vi "Temperature Device (Set).vi"(6 "ISOBUS address":T10=-1 caption="ISOBUS address (-1)", 8 "error in":errorcluster, 10 "Temperature Device Settings":T3, 11 "Mercury Reference In":T11) -> (0 "error out":errorcluster, 2 "Response":T1, 3 "Mercury Reference Out":T11, 4 "Valid?":T2)   [LabVIEW 2013, in "Mercury iXX.lvlib" / "Temperature.lvlib"]
doc: "Set the temperature device configuration."
uses:
  Temperature.lvlib
  Mercury iXX.lvlib
  Private/Controls/Command Verbs.ctl
  Controls/Is Valid LED.ctl
  Controls/Comms Transport Layer.ctl
  Controls/Mercury Reference.ctl
  Controls/Excitation Type.ctl
  Controls/Response String.ctl
  Controls/ISOBus Address.ctl
  Private/Controls/Query Dynamic Reference.ctl
  Controls/Temperature Sensor Type.ctl
  Controls/Excitation Cluster.ctl
  Controls/Calibration Interpolation.ctl
  Controls/Calibration Cluster.ctl
  Controls/Loop Cluster.ctl
  Controls/Temperature Device (Set).ctl
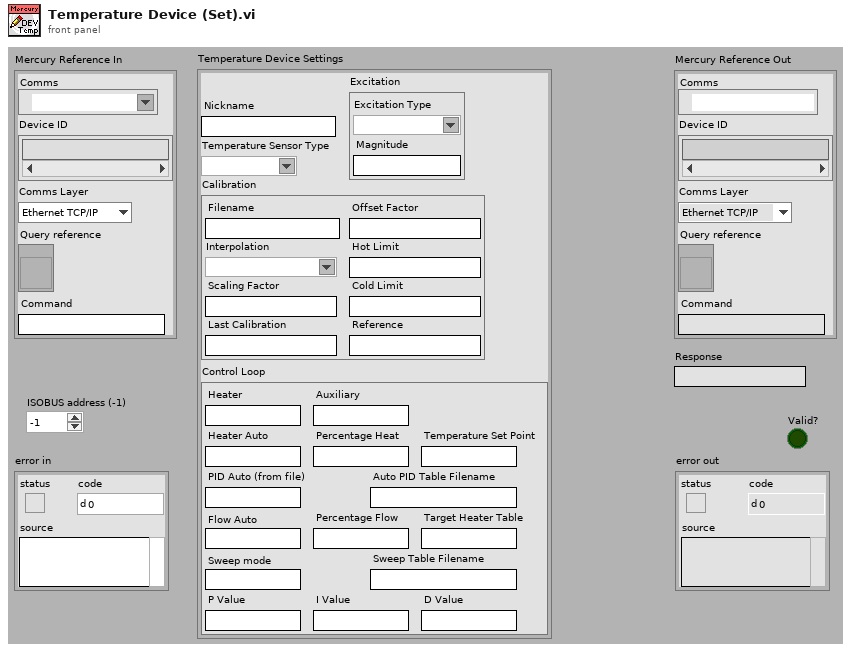
[diagram p1: front panel]
types:
  T1 = typedef "Mercury iXX.lvlib/Response String.ctl" = string
  T2 = typedef "Mercury iXX.lvlib/Is Valid LED.ctl" = bool
  T3 = typedef "Mercury iXX.lvlib/Temperature.lvlib/Temperature Device (Set).ctl" = cluster{"Nickname":string, "Temperature Sensor Type":T4, "Excitation":T5, "Calibration":T7, "Control Loop":T9}
  T4 = typedef "Mercury iXX.lvlib/Temperature.lvlib/Temperature Sensor Type.ctl" = string
  T5 = typedef "Mercury iXX.lvlib/Temperature.lvlib/Excitation Cluster.ctl" = cluster{"Excitation Type":T6, "Magnitude":string}
  T6 = typedef "Mercury iXX.lvlib/Temperature.lvlib/Excitation Type.ctl" = string
  T7 = typedef "Mercury iXX.lvlib/Temperature.lvlib/Calibration Cluster.ctl" = cluster{"Filename":string, "Interpolation":T8, "Scaling Factor":string, "Offset Factor":string, "Hot Limit":string, "Cold Limit":string, "Last Calibration":string, "Reference":string}
  T8 = typedef "Mercury iXX.lvlib/Temperature.lvlib/Calibration Interpolation.ctl" = string
  T9 = typedef "Mercury iXX.lvlib/Temperature.lvlib/Loop Cluster.ctl" = cluster{"Heater":string, "Auxiliary":string, "Heater Auto":string, "Percentage Heat":string, "Temperature Set Point":string, "PID Auto (from file)":string, "P Value":string, "I Value":string, "D Value":string, "Auto PID Table Filename":string, "Flow Auto":string, "Target Heater Table":string, "Sweep mode":string, "Sweep Table Filename":string, "Percentage Flow":string}
  T10 = typedef "Mercury iXX.lvlib/ISOBus Address.ctl" = i32
  T11 = typedef "Mercury iXX.lvlib/Mercury Reference.ctl" = cluster{"Comms":refnum<visa-resource-name>, "Device ID":string[], "Comms Layer":T12, "Command":string, "Query reference":T13}
  T12 = typedef "Mercury iXX.lvlib/Comms Transport Layer.ctl" = enum16{"Ethernet TCP/IP", "USB", "ISOBus - RS-232", "GPIB"}
  T13 = typedef "Mercury iXX.lvlib/Query Dynamic Reference.ctl" = refnum<vi>
  T14 = typedef "Mercury iXX.lvlib/Command Verbs.ctl" = string
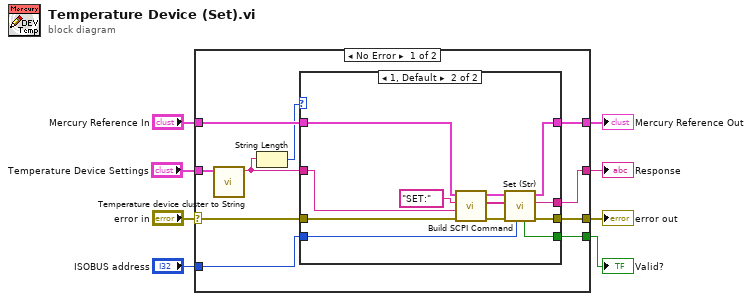
[diagram p0: block diagram]
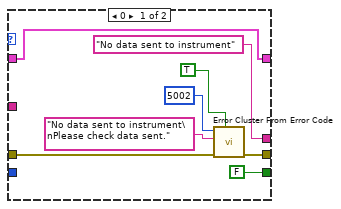
[diagram p2: hidden frame]
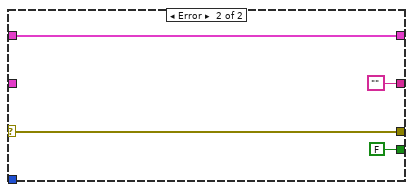
[diagram p3: hidden frame]
diagram:
  n1 = case shown="No Error" "error in" {
    selector: "error in" -> [w16 w41]
    tunnel: "Mercury Reference In" -> [w18 w42]
    tunnel: [w14 w42] -> w7
    tunnel: [w15 w41] -> w6
    tunnel: "ISOBUS address" -> [w17 _]
    tunnel: [w9 ""] -> w2
    tunnel: [w10 FALSE ("Valid?")] -> w3
    tunnel: "Temperature Device Settings" -> [w13 _]
    frame No Error {
      n2 = call "Temperature device cluster to String.vi"("Temperature Device Settings"=w13) -> ("Data to send"=w11:string)  [unwired: 10 out]
      n3 = String Length(string=w11) -> (length=w12:i32)
      n4 = case shown="1, Default" w12 {
        tunnel: w18 -> [w26 w28]
        tunnel: w17 -> [_ w30]
        tunnel: w16 -> [w24 w29]
        tunnel: [w25 w31] -> w15
        tunnel: [w26 w32] -> w14
        tunnel: w11 -> [_ w27]
        tunnel: [T2 FALSE ("Valid?") w34] -> w10
        tunnel: ["No data sent to instrument" ("Data") w33] -> w9
        frame 0 {
          n5 = call <vilib>:"Error Cluster From Error Code.vi"("show call chain? (False)"=TRUE, "error in (no error)"=w24, "error message (\"\")"="No data sent to instrument\nPlease check data sent." ("error message (\"\")"), "error code (0)"=5002) -> ("error out"=w25:errorcluster)  [unwired: 5 out]
        }
        frame 1, Default {
          n6 = call "Build SCPI Command.vi"("error in"=w29, "Noun(s)"=w27, "Verb"=T14 "SET:", "Mercury Reference In"=w28) -> ("error out"=w38:errorcluster, "SCPI Message(s)"=w37:string[], "Mercury Reference Out"=w36:T11)  [unwired: 5 out]
          n7 = call "Set (Str).vi"("ISOBUS address"=w30, "error in"=w38, "SCPI Message(s)"=w37, "Mercury Reference In"=w36) -> ("error out"=w31:errorcluster, "Response"=w33:T1, "Mercury Reference Out"=w32:T11, "Valid?"=w34:T2)  [unwired: 1 in, 3 out]
        }
      }
    }
    frame Error {
    }
  }
  "Mercury Reference Out" <- w7
  "error out" <- w6
  "Valid?" <- w3
  "Response" <- w2
